vi "RT 2.0.vi"() -> ()   [LabVIEW 2014]
uses:
  FPGA Bitfiles/Parking States Indicators.ctl
  FPGA Bitfiles/Parking States.ctl
  <vilib>/FPGAPlugInAG/myRIO-1950/niLvFpga_Open_myRIO-1950.vi
  <vilib>/rvi/interface/common/dynamic/niFpgaDynamicAddResources.vi
  <vilib>/FPGAPlugInAG/Dynamic/niLvFpga_Close_Dynamic.vi
  <vilib>/rvi/interface/nirviOpenFPGA/nirviOpenFPGA.xnode
  FPGA Bitfiles/SensorMain_FPGATarget_ParallaxPING)))(_3ylNEQ+tG2M.lvbitx
  <instrlib>/Parallax PING)))/FPGA Example/Parallax PING))) (FPGA).vi
  <vilib>/rvi/interface/nirviCloseFPGA/nirviCloseFPGA.xnode
panel:
  out "Output Cluster":T1={"myRio / RC Control"=FALSE, "Right Radio"=FALSE, "Left Radio"=FALSE, "Front"=37.140828371047974, "Front Side"=39.974039793014526, "Back Side"=42.377978563308716, "Back"=166.97952270507812, "Front Speed"=17, "Back Speed"=17} {"Back Speed" scale=0.0..50.0; "Front Speed" scale=0.0..50.0}
  out "Cluster":T2
  in  "stop":bool
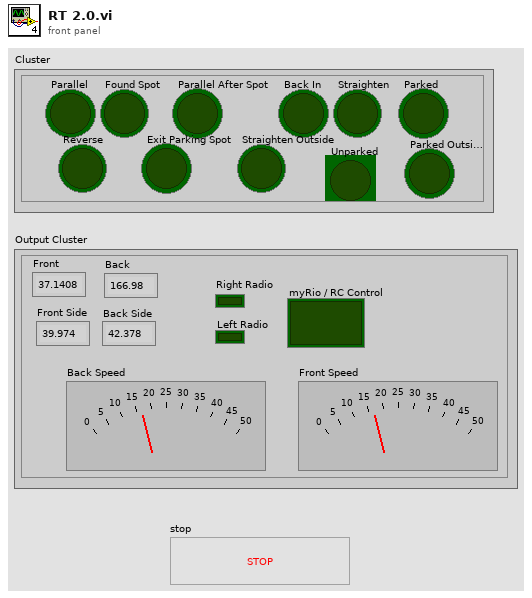
[diagram p1: front panel]
types:
  T1 = cluster{"myRio / RC Control":bool, "Right Radio":bool, "Left Radio":bool, "Front":dbl, "Front Side":dbl, "Back Side":dbl, "Back":dbl, "Front Speed":u32, "Back Speed":u32}
  T2 = typedef "Parking States Indicators.ctl" = cluster{"Parallel":bool, "Found Spot":bool, "Parallel After Spot":bool, "Back In":bool, "Straighten":bool, "Parked":bool, "Reverse":bool, "Exit Parking Spot":bool, "Straighten Outside":bool, "Unparked":bool, "Parked Outside":bool}
  T3 = typedef "Parking States.ctl" = enum16{"Drive", "Parallel", "Found Spot", "Parallel After Spot", "Back In", "Straighten", "Parked", "Reverse", "Exit Parking Spot", "Straighten Outside", "Unparked", "Parked Outside"}
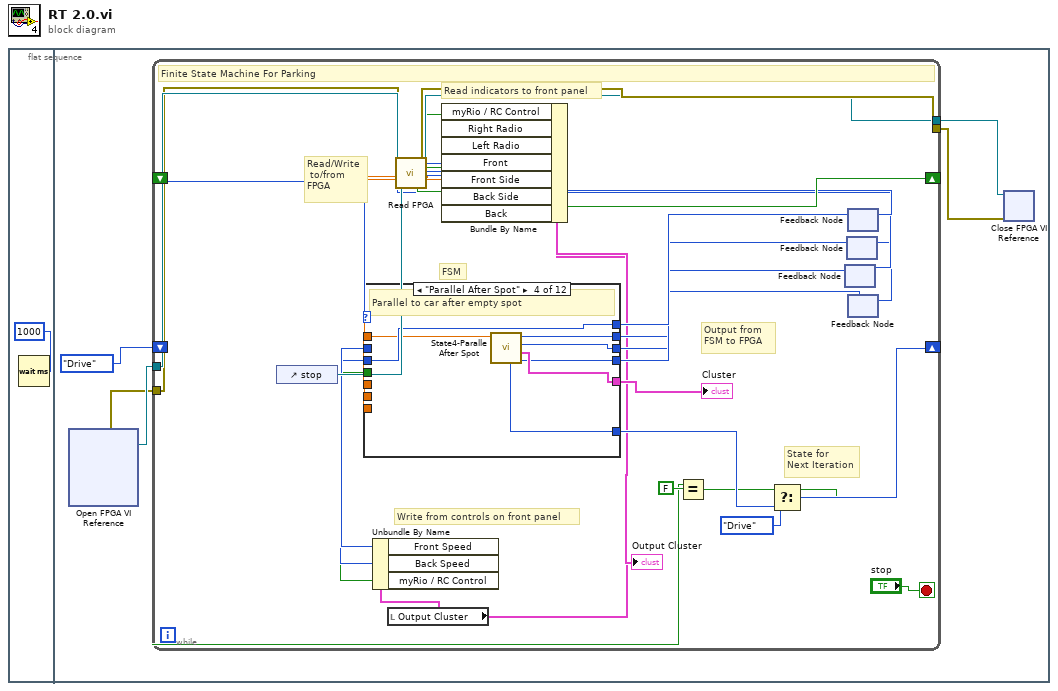
[diagram p0: block diagram]
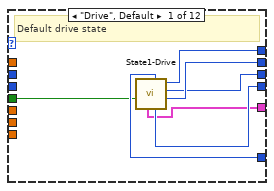
[diagram p2: hidden frame]
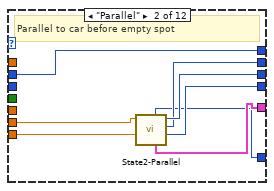
[diagram p3: hidden frame]
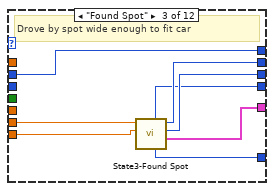
[diagram p4: hidden frame]
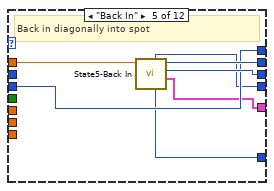
[diagram p5: hidden frame]
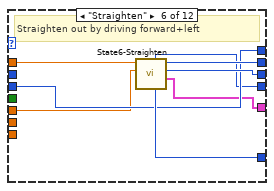
[diagram p6: hidden frame]
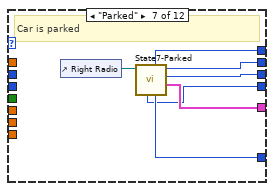
[diagram p7: hidden frame]
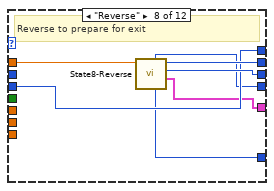
[diagram p8: hidden frame]
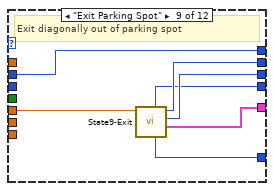
[diagram p9: hidden frame]
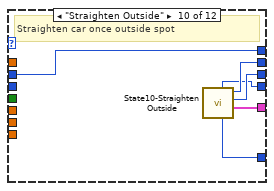
[diagram p10: hidden frame]
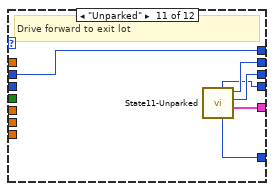
[diagram p11: hidden frame]
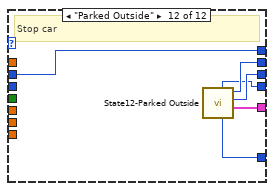
[diagram p12: hidden frame]
diagram:
  n1 = flat-sequence {
    frame #0 {
      n2 = Wait (ms)(milliseconds to wait=u32 1000) -> ()  [unwired: 1 out]
    }
    frame #1 {
      n3 = xnode "Open FPGA VI Reference"() -> ("FPGA VI Reference Out"=w6:refnum<k20>, "error out"=w5:errorcluster)  [unwired: 2 in]
      n4 = while {
        tunnel: w6 -> [w41]
        tunnel: w5 -> [w40]
        tunnel: [w39] -> w4
        tunnel: [w38] -> w3
        shift-right: [w34] -> _
        shift-left: Parking_States."Drive" -> [w36]
        shift-right: [w31] -> _
        shift-left: _ -> [w30]
        stop <- "stop" stop-if-true
        # "State for\nNext Iteration"
        # "Output from \nFSM to FPGA"
        # "Read/Write\n to/from\nFPGA"
        # "FSM"
        # "Write from controls on front panel"
        # "Read indicators to front panel"
        # "Finite State Machine For Parking"
        n5 = control-ref of="stop"() -> (w27:refnum<vi>)
        n6 = local read "Output Cluster"() -> (w15:T1)
        n7 = Unbundle By Name(w15) -> ("Front Speed"=w14:u32, "Back Speed"=w13:u32, "myRio / RC Control"=w12:bool)
        n8 = Equal?(x=w30, y=FALSE) -> (x = y?=w32:bool)
        n9 = feedback #1() -> (w23:u32)  [unwired: 1 in]
        n10 = feedback #2() -> (w21:enum16{"Left", "Right", "Stop"})  [unwired: 1 in]
        n11 = feedback #3() -> (w25:u32)  [unwired: 1 in]
        n12 = feedback #4() -> (w7:enum16{"Forward", "Backward", "Stop"})  [unwired: 1 in]
        n13 = call "Read FPGA.vi"("Refnum in"=w41, "Front/Back Speed"=w25, "Front/Back in"=w7, "Left/Right Speed"=w23, "Left/Right"=w21, "error in (no error)"=w40, "reference"=w27) -> ("Front"=w10:dbl, "myRio / RC Control"=w18:bool, "Front Side"=w9:dbl, "Right Radio"=w19:bool, "myRio / RC Control 2"=w31:bool, "Refnum out"=w38:refnum<k20>, "Left Radio"=w17:bool, "Back Side"=w8:dbl, "Back"=w11:dbl, "error out"=w39:errorcluster)  [unwired: 6 in, 5 out]
        n14 = case shown="\"Parallel After Spot\"" w36 {
          tunnel: [w44 w49 w64 w68 w75 w85 w91 w97 w104 w110 w117 w125] -> w35
          tunnel: [w45 w51 w57 w65 w72 w79 w88 w94 w101 w108 w114 w120] -> w24
          tunnel: [w48 w52 w63 w71 w78 w86 w93 w100 w106 w112 w119 w123] -> w22
          tunnel: [w47 w53 w62 w70 w77 w84 w92 w99 w105 w113 w118 w122] -> w20
          tunnel: [w46 w56 w61 w69 w76 w83 w87 w98 w107 w111 w116 w124] -> w26
          tunnel: w14 -> [_ w56 w61 _ _ _ _ _ w107 w111 w116 w124]
          tunnel: w13 -> [_ _ _ w69 w76 w83 _ w98 _ _ _ _]
          tunnel: [w43 w50 w58 w66 w73 w80 w90 w95 w102 w109 w115 w121] -> w28
          tunnel: w9 -> [_ w55 w60 _ _ _ _ _ _ _ _ _]
          tunnel: w8 -> [_ w54 w59 _ _ _ _ _ _ _ _ _]
          tunnel: w11 -> [_ _ _ w67 w74 w81 _ w96 _ _ _ _]
          tunnel: w10 -> [_ _ _ _ _ w82 _ _ w103 _ _ _]
          tunnel: w12 -> [w42 _ _ _ _ _ _ _ _ _ _ _]
          frame "Drive", Default {
            # "Default drive state"
            n15 = call "State1-Drive.vi"("Boolean"=w42) -> ("Left/Right"=w48:enum16{"Left", "Right", "Stop"}, "Front/Back 2"=w47:enum16{"Forward", "Backward", "Stop"}, "Front/Back Speed"=w46:u32, "Left/Right Speed"=w45:u32, "Enum"=w44:T3, "Cluster"=w43:T2)  [unwired: 5 in]
          }
          frame "Parallel" {
            # "Parallel to car before empty spot"
            n16 = call "State2-Parallel.vi"("Numeric 7"=w54, "Numeric in"=w55) -> ("Init Left/Right Speed 3"=w51:u32, "Left/Right"=w52:enum16{"Left", "Right", "Stop"}, "Front/Back 2"=w53:enum16{"Forward", "Backward", "Stop"}, "Cluster"=w50:T2, "Enum"=w49:T3)  [unwired: 5 in]
          }
          frame "Found Spot" {
            # "Drove by spot wide enough to fit car"
            n17 = call "State3-Found Spot.vi"("Numeric"=w59, "Numeric 2"=w60) -> ("Cluster"=w58:T2, "Front/Back 2"=w62:enum16{"Forward", "Backward", "Stop"}, "Left/Right"=w63:enum16{"Left", "Right", "Stop"}, "Enum"=w64:T3, "Left/Right Speed"=w57:u32)  [unwired: 5 in]
          }
          frame "Parallel After Spot" {
            # "Parallel to car after empty spot"
            n18 = call "State4-Paralle After Spot.vi"("Numeric"=w67) -> ("Cluster"=w66:T2, "Front/Back 2"=w70:enum16{"Forward", "Backward", "Stop"}, "Left/Right"=w71:enum16{"Left", "Right", "Stop"}, "Enum"=w68:T3, "Left/Right Speed"=w65:u32)  [unwired: 6 in]
          }
          frame "Back In" {
            # "Back in diagonally into spot"
            n19 = call "State5-Back In.vi"("Numeric"=w74) -> ("Cluster"=w73:T2, "Front/Back 2"=w77:enum16{"Forward", "Backward", "Stop"}, "Left/Right"=w78:enum16{"Left", "Right", "Stop"}, "Enum"=w75:T3, "Left/Right Speed"=w72:u32)  [unwired: 6 in]
          }
          frame "Straighten" {
            # "Straighten out by driving forward+left"
            n20 = call "State6-Straighten.vi"("Numeric 2"=w82, "Numeric"=w81) -> ("Cluster"=w80:T2, "Front/Back 2"=w84:enum16{"Forward", "Backward", "Stop"}, "Left/Right"=w86:enum16{"Left", "Right", "Stop"}, "Enum"=w85:T3, "Left/Right Speed"=w79:u32)  [unwired: 5 in]
          }
          frame "Parked" {
            # "Car is parked"
            n21 = control-ref of="Right Radio"() -> (w89:refnum<vi>)
            n22 = call "State7-Parked.vi"("Boolean in"=w89) -> ("Cluster"=w90:T2, "Front/Back 2"=w92:enum16{"Forward", "Backward", "Stop"}, "Left/Right"=w93:enum16{"Left", "Right", "Stop"}, "Enum"=w91:T3, "Back Speed"=w87:u32, "Left/Right Speed"=w88:u32)  [unwired: 5 in]
          }
          frame "Reverse" {
            # "Reverse to prepare for exit"
            n23 = call "State8-Reverse.vi"("Numeric"=w96) -> ("Cluster"=w95:T2, "Front/Back 2"=w99:enum16{"Forward", "Backward", "Stop"}, "Left/Right"=w100:enum16{"Left", "Right", "Stop"}, "Enum"=w97:T3, "Left/Right Speed"=w94:u32)  [unwired: 6 in]
          }
          frame "Exit Parking Spot" {
            # "Exit diagonally out of parking spot"
            n24 = call "State9-Exit.vi"("Numeric"=w103) -> ("Cluster"=w102:T2, "Front/Back 2"=w105:enum16{"Forward", "Backward", "Stop"}, "Left/Right"=w106:enum16{"Left", "Right", "Stop"}, "f"=w104:T3, "Left/Right Speed"=w101:u32)  [unwired: 6 in]
          }
          frame "Straighten Outside" {
            # "Straighten car once outside spot"
            n25 = call "State10-Straighten Outside.vi"() -> ("Cluster"=w109:T2, "Front/Back 2"=w113:enum16{"Forward", "Backward", "Stop"}, "Left/Right"=w112:enum16{"Left", "Right", "Stop"}, "f"=w110:T3, "Left/Right Speed"=w108:u32)  [unwired: 7 in]
          }
          frame "Unparked" {
            # "Drive forward to exit lot"
            n26 = call "State11-Unparked.vi"() -> ("Cluster"=w115:T2, "Front/Back 2"=w118:enum16{"Forward", "Backward", "Stop"}, "Left/Right"=w119:enum16{"Left", "Right", "Stop"}, "f"=w117:T3, "Left/Right Speed"=w114:u32)  [unwired: 7 in]
          }
          frame "Parked Outside" {
            # "Stop car"
            n27 = call "State12-Parked Outside.vi"() -> ("Cluster"=w121:T2, "Front/Back 2"=w122:enum16{"Forward", "Backward", "Stop"}, "Left/Right"=w123:enum16{"Left", "Right", "Stop"}, "f"=w125:T3, "Left/Right Speed"=w120:u32)  [unwired: 7 in]
          }
        }
        "Cluster" <- w28
        n28 = Bundle By Name(cluster=w15, "myRio / RC Control"=w18, "Right Radio"=w19, "Left Radio"=w17, "Front"=w10, "Front Side"=w9, "Back Side"=w8, "Back"=w11) -> (→"Output Cluster":T1)
        n29 = Select(t=Parking_States."Drive", s=w32, f=w35) -> (s? t:f=w34:T3)
        n30 = feedback-in #1(w24) -> ()
        n31 = feedback-in #2(w22) -> ()
        n32 = feedback-in #3(w26) -> ()
        n33 = feedback-in #4(w20) -> ()
      }
      n34 = xnode "Close FPGA VI Reference"("FPGA VI Reference In"=w3, "error in"=w4) -> ()  [unwired: 1 out]
    }
  }
